vi "4.6.4.vi"() -> ()   [LabVIEW 2017]
panel:
  in  "停止":bool
  out "结果":dbl
  in  "y":dbl
  in  "x":dbl
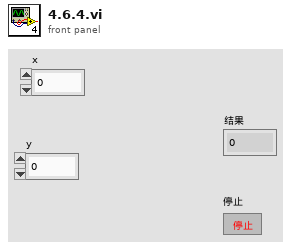
[diagram p1: front panel]
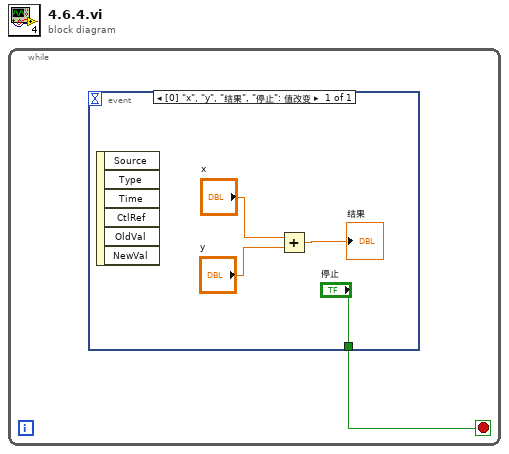
[diagram p0: block diagram]
diagram:
  n1 = while {
    stop <- w1 stop-if-true
    n2 = event shown="[0] \"x\", \"y\", \"结果\", \"停止\": 值改变" {
      selector: _ -> [_]
      dyn-events: _ -> [_]
      timeout: _ -> [_]
      tunnel: ["停止"] -> w1
      event "x", "y", "结果", "停止": Value Change {
        n3 = event-data() -> ()  [unwired: 1 in, 6 out]
        n4 = Add(x="x", y="y") -> (x+y=→"结果":dbl)
      }
    }
  }
